vi "Add New Headers.vi"(8 "error in (no error)":errorcluster, 10 "Incoming Headers[]":string[](array[string]), 11 "Existing Headers[]":string[](array[string])) -> (0 "error out":errorcluster, 3 "Headers[] Out":string[](array[string]))   [LabVIEW 2014, in "SLL Spreadsheet.lvlib" / "SLL CSV Logger.lvclass"]
doc: "Supports writing of 2D string with new line & comma to a spreadsheet file, which are not supported by LabVIEW's builtin function.\n\nIts functionality is similar to how Excel does it - it adds double quotes to cells which contains new line character, comma and double quotes. If the cell already has double quotes, it escapes it with one more double quotes."
uses:
  SLL CSV Logger.lvclass
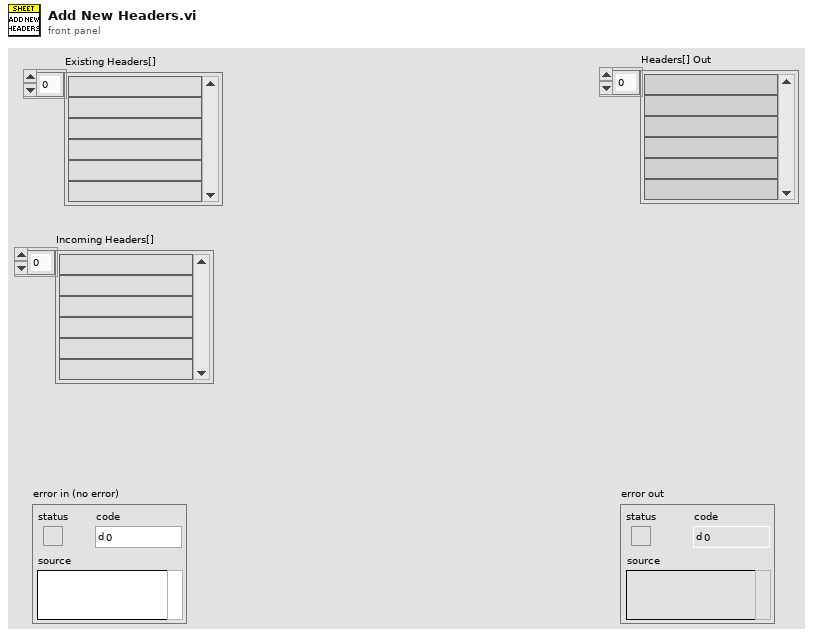
[diagram p1: front panel]
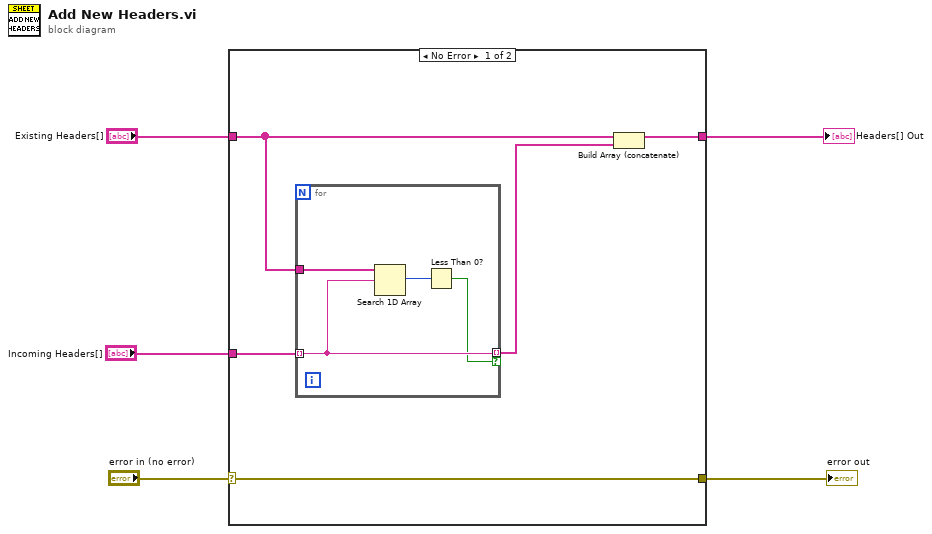
[diagram p0: block diagram]
diagram:
  n1 = case shown="No Error" "error in (no error)" {
    selector: "error in (no error)" -> [w7 w16]
    tunnel: [w7 w16] -> w5
    tunnel: "Existing Headers[]" -> [w9 w15]
    tunnel: "Incoming Headers[]" -> [w10 _]
    tunnel: [w6 w15] -> w1
    frame No Error {
      n2 = for {
        tunnel: w10 -> [w12] mode=indexing
        tunnel: w9 -> [w14]
        tunnel: [w12] -> w8 mode=indexing if=w11
        n3 = Search 1D Array(1D array=w14, element=w12) -> (index of element=w13:i32)  [unwired: 1 in]
        n4 = Less Than 0?(x=w13) -> (x < 0?=w11:bool)
      }
      n5 = Build Array (concatenate)(w9, w8) -> (w6:string[])
    }
    frame Error {
    }
  }
  "error out" <- w5
  "Headers[] Out" <- w1
